vi "CRYReport Part ObjectChange Event Callback.vi"(4 "TXTextControl":refnum<k7>, 6 "Control Ref":refnum<k7>, 7 "Event Common Data":T1) -> ()   [LabVIEW 2013]
uses:
  CRYProject/CRYProject Editor Global.vi
  CRYReport Global.vi
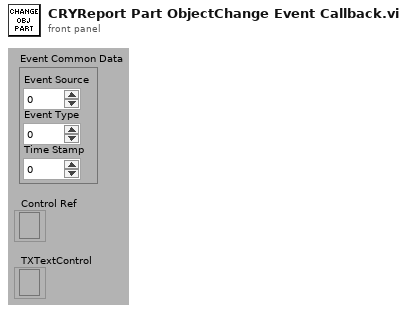
[diagram p1: front panel]
types:
  T1 = cluster{"Event Source":i32, "Event Type":u32, "Time Stamp":u32}
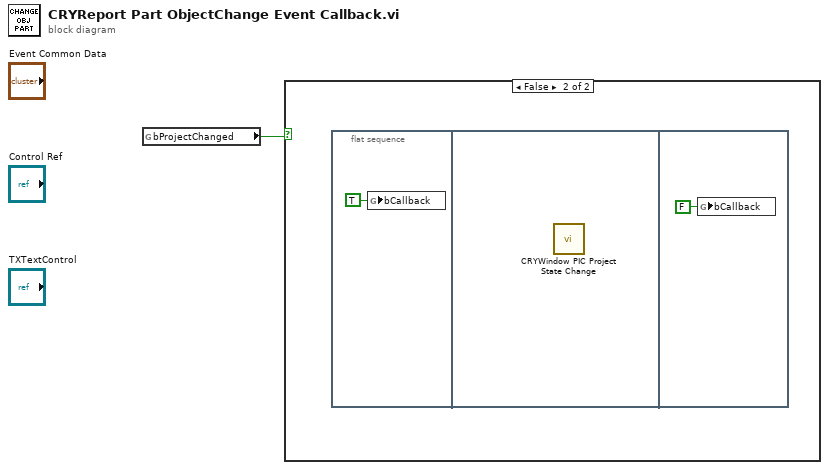
[diagram p0: block diagram]
diagram:
  n1 = global read "CRYProject Editor Global.vi" "bProjectChanged"() -> (w1:bool)
  n2 = case shown="False" w1 {
    frame True {
    }
    frame False {
      n3 = flat-sequence {
        frame #0 {
          n4 = global write "CRYReport Global.vi" "bCallback"(TRUE ("bCallback")) -> ()
        }
        frame #1 {
          n5 = call "CRYWindow PIC Project State Change.vi"() -> ()  [unwired: 12 in]
        }
        frame #2 {
          n6 = global write "CRYReport Global.vi" "bCallback"(FALSE ("bCallback")) -> ()
        }
      }
    }
  }
